vi "MORSE CODE PROJECT COMPLETE.vi"() -> ()   [LabVIEW 2012]
uses:
  <vilib>/Utility/file.llb/Read From Spreadsheet File (string).vi
panel:
  in  "Device Name":tag="Dev1"
  in  "Morse Code Lookup Table File Path":path
  in  "STOP PROGRAM":bool
  in  "Lookup Table":T1
  in  "?":T2(tab)
  out "Telegraph Mode":bool
  out "Light Output":bool
  out "Morse Code Translation":string
  in  "Text Input":string
  in  "Transmit Button":bool
  in  "Dot Speed":dbl(slide) step=5.0 scale=100.0..300.0 scale format="%#_5g"
  in  "RESET TEXT":bool
  out "Translated":string
  out "Waveform Chart":dbl(graph)
  in  "Rate":dbl=1000.0
  in  "Samples":i32=1000
  out "LIVE Decoded Morse Code":string
  in  "Array 2":string[](array[string])
  in  "Array":string[](array[string])
  out "[DEBUG]\nText Indicator":string[](array[string])
  out "[DEBUG]\nIndex of Last Element":i32
  out "[DEBUG] \nMorse Code":string[](array[string])
  out "[DEBUG]\nString":string
  out "Sample Number":dbl
  out "[DEBUG]\nMorse Code Words":string[](array[string])
  in  "Array 3":string[](array[string])
  out "[DEBUG]\nMorse Code Letters":string[](array[string])
  # "Recommended\nSetting:\n\n1. Rate (10000) \n2. Samples (10)"
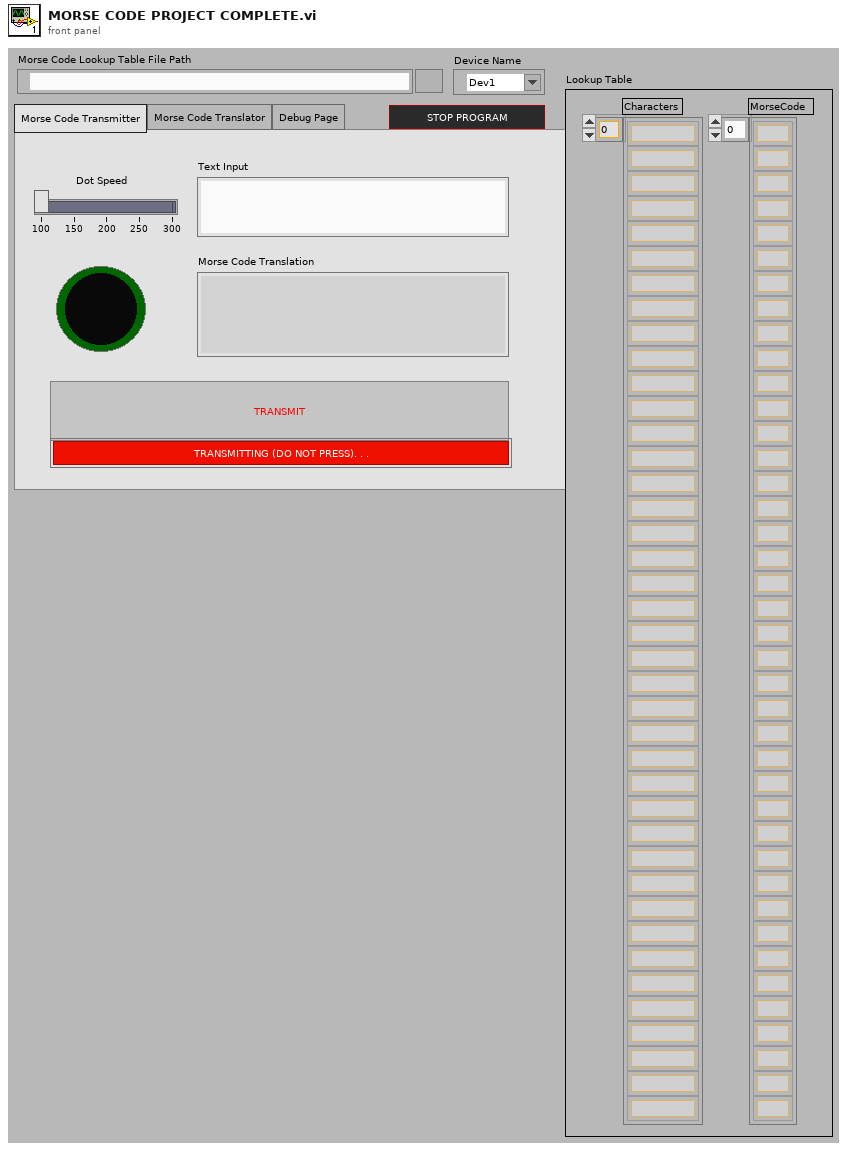
[diagram p1: front panel]
types:
  T1 = cluster{"Characters":string[], "MorseCode":string[]}
  T2 = enum32{"Morse Code Transmitter", "Morse Code Translator", "Debug Page"}
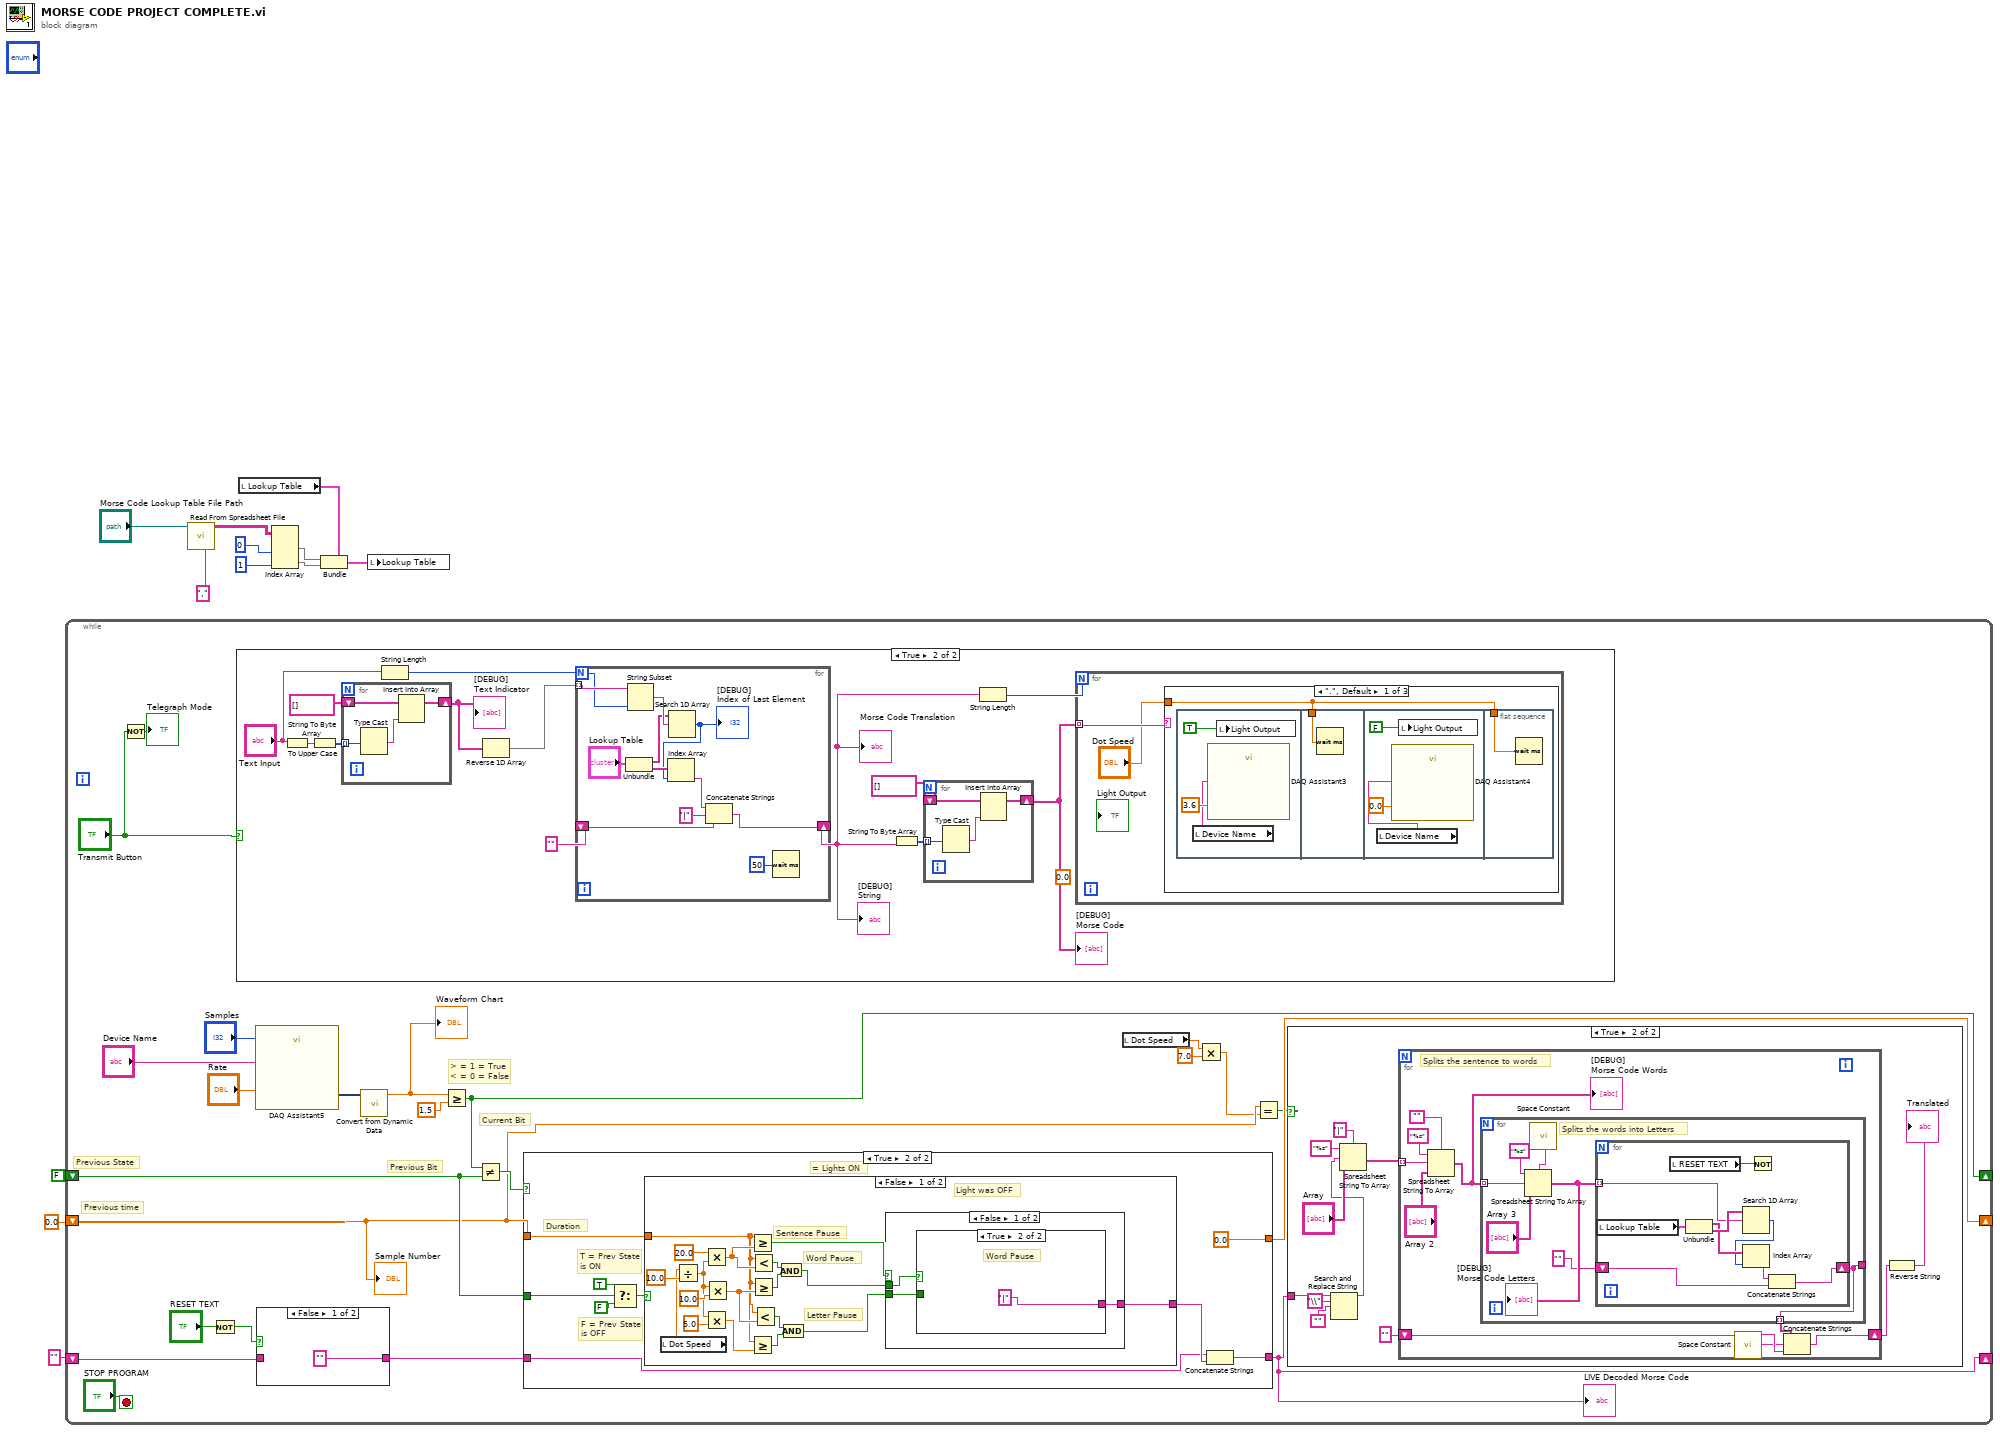
[diagram p0: block diagram]
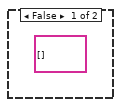
[diagram p2: hidden frame]
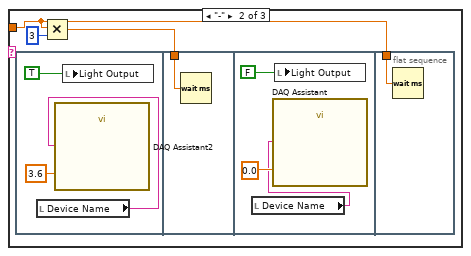
[diagram p5: hidden frame]
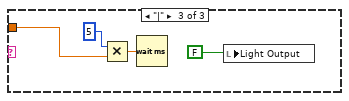
[diagram p6: hidden frame]
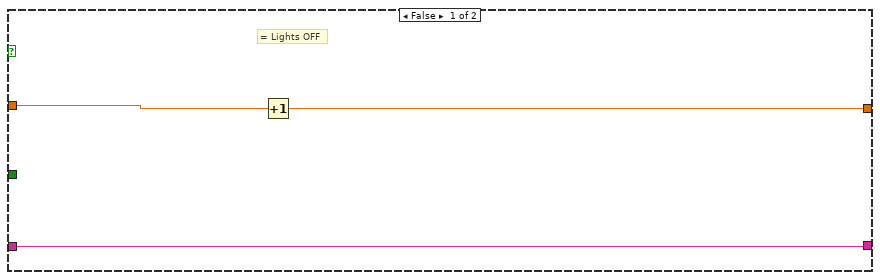
[diagram p7: hidden frame]
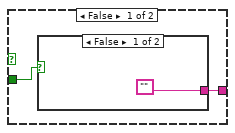
[diagram p8: hidden frame]
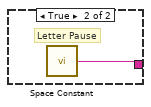
[diagram p9: hidden frame]
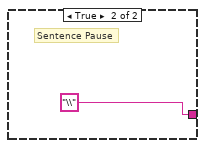
[diagram p10: hidden frame]
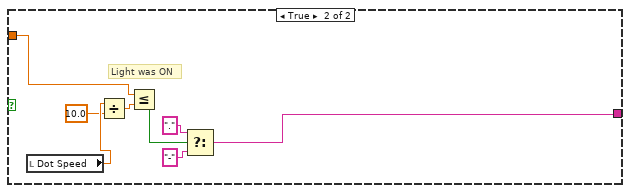
[diagram p11: hidden frame]
diagram:
  n1 = while {
    shift-right: [w29] -> _
    shift-left: FALSE -> [w27]
    shift-right: [w28] -> _
    shift-left: 0.0 -> [w14]
    shift-right: [w18] -> _
    shift-left: "" -> [w21]
    stop <- "STOP PROGRAM" stop-if-true
    # "Previous Bit"
    # "Current Bit"
    # "> = 1 = True\n< = 0 = False"
    # "Previous time"
    # "Previous State"
    n2 = Not(x="Transmit Button") -> (.not. x?=→"Telegraph Mode":bool)
    n3 = Not(x="RESET TEXT") -> (.not. x?=w19:bool)
    n4 = case shown="True" "Transmit Button" {
      frame False {
      }
      frame True {
        (unwired) 0.0
        n5 = To Upper Case(1:"Text Input") -> (0:w84:string)
        n6 = String To Byte Array(string=w84) -> (unsigned byte array=w83:u8[])
        n7 = for {
          tunnel: w83 -> [w120] mode=indexing
          shift-right: [w118] -> w80
          shift-left: string[] [] -> [w119]
          n8 = Type Cast(x=w120) -> (*(type *) &x=w117:string)  [unwired: 1 in]
          n9 = Insert Into Array(array=w119, new element=w117) -> (w118:string[])  [unwired: 1 in]
        }
        "[DEBUG]\nText Indicator" <- w80
        n10 = String Length(string="Text Input") -> (length=w86:i32)
        n11 = Reverse 1D Array(array=w80) -> (reversed array=w81:string[])
        n12 = for {
          N: w86 -> [w125]
          tunnel: w81 -> [w132] mode=indexing
          shift-right: [w122] -> w76
          shift-left: "" -> [w130]
          n13 = Unbundle("Lookup Table") -> ("Characters"=w129:string[], "MorseCode"=w128:string[])
          n14 = String Subset(string=w132, length (rest)=w125) -> (substring=w131:string)  [unwired: 1 in]
          n15 = Search 1D Array(1D array=w129, element=w131) -> (index of element=w124:i32)  [unwired: 1 in]
          "[DEBUG]\nIndex of Last Element" <- w124
          n16 = Index Array(array=w128, index=w124) -> (element=w126:string)
          n17 = Concatenate Strings(w126, "|", w130) -> (w122:string)
          n18 = Wait (ms)(milliseconds to wait=u32 50) -> ()  [unwired: 1 out]
        }
        "Morse Code Translation" <- w76
        "[DEBUG]\nString" <- w76
        n19 = String To Byte Array(string=w76) -> (unsigned byte array=w78:u8[])
        n20 = for {
          tunnel: w78 -> [w116] mode=indexing
          shift-right: [w114] -> w77
          shift-left: string[] [] -> [w115]
          n21 = Type Cast(x=w116) -> (*(type *) &x=w113:string)  [unwired: 1 in]
          n22 = Insert Into Array(array=w115, new element=w113) -> (w114:string[])  [unwired: 1 in]
        }
        "[DEBUG] \nMorse Code" <- w77
        n23 = String Length(string=w76) -> (length=w75:i32)
        n24 = for {
          N: w75 -> [_]
          tunnel: w77 -> [w88] mode=indexing
          n25 = case shown="\".\", Default" w88 {
            tunnel: "Dot Speed" -> [w89 w98 w110]
            frame ".", Default {
              n26 = flat-sequence {
                tunnel: w89 -> [w93]
                tunnel: w89 -> [w97]
                frame #0 {
                  n27 = local read "Device Name"() -> (w90:tag)
                  n28 = call "DAQ Assistant3"("data"=3.6, "device name"=w90) -> ()  [unwired: 16 in, 2 out]
                  n29 = local write "Light Output"(TRUE) -> ()
                }
                frame #1 {
                  n30 = Wait (ms)(milliseconds to wait=w93) -> ()  [unwired: 1 out]
                }
                frame #2 {
                  n31 = local read "Device Name"() -> (w94:tag)
                  n32 = call "DAQ Assistant4"("data"=0.0, "device name"=w94) -> ()  [unwired: 16 in, 2 out]
                  n33 = local write "Light Output"(FALSE) -> ()
                }
                frame #3 {
                  n34 = Wait (ms)(milliseconds to wait=w97) -> ()  [unwired: 1 out]
                }
              }
            }
            frame "-" {
              n35 = flat-sequence {
                tunnel: w99 -> [w104]
                tunnel: w98 -> [w108]
                frame #0 {
                  n36 = local read "Device Name"() -> (w101:tag)
                  n37 = call "DAQ Assistant2"("data"=3.6 ("t"), "device name"=w101) -> ()  [unwired: 16 in, 2 out]
                  n38 = local write "Light Output"(TRUE) -> ()
                }
                frame #1 {
                  n39 = Wait (ms)(milliseconds to wait=w104) -> ()  [unwired: 1 out]
                }
                frame #2 {
                  n40 = local read "Device Name"() -> (w105:tag)
                  n41 = call "DAQ Assistant"("data"=0.0 ("f"), "device name"=w105) -> ()  [unwired: 16 in, 2 out]
                  n42 = local write "Light Output"(FALSE) -> ()
                }
                frame #3 {
                  n43 = Wait (ms)(milliseconds to wait=w108) -> ()  [unwired: 1 out]
                }
              }
              n44 = Multiply(x=w98, y=3) -> (x*y=w99:dbl)
            }
            frame "|" {
              n45 = Multiply(x=5, y=w110) -> (x*y=w112:dbl)
              n46 = Wait (ms)(milliseconds to wait=w112) -> ()  [unwired: 1 out]
              n47 = local write "Light Output"(FALSE ("Time has Elapsed")) -> ()
            }
          }
        }
      }
    }
    n48 = call "DAQ Assistant5"("rate"="Rate", "number of samples"="Samples", "device name"="Device Name") -> ("data"=w31:dynamicdata)  [unwired: 14 in, 2 out]
    n49 = case shown="False" w19 {
      tunnel: w21 -> [_ w73]
      tunnel: ["" w73] -> w22
      frame False {
      }
      frame True {
      }
    }
    n50 = call "Convert from Dynamic Data"("Dynamic Data Type"=w31) -> ("Scalar"=w32:dbl)  [unwired: 3 in]
    "Waveform Chart" <- w32
    n51 = Greater Or Equal?(x=w32, y=1.5) -> (x >= y?=w29:bool)
    n52 = Not Equal?(x=w29, y=w27) -> (x != y?=w30:bool)
    n53 = case shown="True" w30 {
      tunnel: w14 -> [w135 w139]
      tunnel: [w133 0.0] -> w28
      tunnel: w27 -> [_ w144]
      tunnel: [w134 w140] -> w18
      tunnel: w22 -> [w134 w136]
      frame False {
        # "= Lights OFF"
        n54 = Increment(x=w135) -> (x+1=w133:dbl)
      }
      frame True {
        # "F = Prev State\nis OFF"
        # "T = Prev State\nis ON"
        # "Duration"
        # "= Lights ON"
        n55 = Select(t=TRUE, s=w144, f=FALSE) -> (s? t:f=w141:bool)
        n56 = case shown="False" w141 {
          tunnel: [w148 w176] -> w137
          tunnel: w139 -> [w145 w175]
          frame False {
            # "Letter Pause"
            # "Word Pause"
            # "Sentence Pause"
            # "Light was OFF"
            n57 = local read "Dot Speed"() -> (w159:dbl)
            n58 = Divide(x=w159, y=10.0) -> (x/y=w146:dbl)
            n59 = Multiply(x=20.0, y=w146) -> (x*y=w155:dbl)
            n60 = Multiply(x=w146, y=5.0 ("x")) -> (x*y=w153:dbl)
            n61 = Multiply(x=w146, y=10.0 ("x")) -> (x*y=w154:dbl)
            n62 = Greater Or Equal?(x=w145, y=w155) -> (x >= y?=w150:bool)
            n63 = Greater Or Equal?(x=w145, y=w153) -> (x >= y?=w151:bool)
            n64 = Less?(x=w145, y=w155) -> (x < y?=w162:bool)
            n65 = Greater Or Equal?(x=w145, y=w154) -> (x >= y?=w161:bool)
            n66 = Less?(x=w145, y=w154) -> (x < y?=w152:bool)
            n67 = And(x=w162, y=w161) -> (x .and. y?=w149:bool)
            n68 = And(x=w152, y=w151) -> (x .and. y?=w147:bool)
            n69 = case shown="False" w150 {
              tunnel: w149 -> [w165 _]
              tunnel: [w164 "\\"] -> w148
              tunnel: w147 -> [w163 _]
              frame False {
                n70 = case shown="True" w165 {
                  tunnel: [w167 "|"] -> w164
                  tunnel: w163 -> [w166 _]
                  frame False {
                    n71 = case shown="False" w166 {
                      tunnel: ["" w169] -> w167
                      frame False {
                      }
                      frame True {
                        # "Letter Pause"
                        n72 = call <vilib>:"Space Constant.vi"() -> ("String"=w169:string)
                      }
                    }
                  }
                  frame True {
                    # "Word Pause"
                  }
                }
              }
              frame True {
                # "Sentence Pause"
              }
            }
          }
          frame True {
            # "Light was ON"
            n73 = local read "Dot Speed"() -> (w173:dbl)
            n74 = Divide(x=w173, y=10.0) -> (x/y=w174:dbl)
            n75 = Less Or Equal?(x=w175, y=w174) -> (x <= y?=w179:bool)
            n76 = Select(t=".", s=w179, f="-") -> (s? t:f=w176:string)
          }
        }
        n77 = Concatenate Strings(w136, w137) -> (w140:string)
      }
    }
    "LIVE Decoded Morse Code" <- w18
    n78 = local read "Dot Speed"() -> (w16:dbl)
    n79 = Multiply(x=w16, y=7.0 ("x")) -> (x*y=w13:dbl)
    n80 = Equal?(x=w14, y=w13) -> (x = y?=w17:bool)
    n81 = case shown="True" w17 {
      tunnel: w18 -> [_ w42]
      frame False {
        (unwired) string[][] [] ("Array 2")
      }
      frame True {
        n82 = Search and Replace String(input string=w42, search string="\\", replace string="") -> (result string=w39:string)  [unwired: 5 in, 3 out]
        n83 = Spreadsheet String To Array(delimiter (Tab)="|" ("regular expression"), format string="%s", spreadsheet string=w39, array type (2D Dbl)="Array") -> (array=w45:string[])
        n84 = for {
          tunnel: w45 -> [w53] mode=indexing
          shift-right: [w50] -> w38
          shift-left: "" -> [w48]
          # "Splits the sentence to words"
          n85 = Spreadsheet String To Array(delimiter (Tab)="", format string="%s", spreadsheet string=w53, array type (2D Dbl)="Array 2") -> (array=w51:string[])
          "[DEBUG]\nMorse Code Words" <- w51
          n86 = for {
            tunnel: w51 -> [w59] mode=indexing
            tunnel: [w57] -> _
            tunnel: [w57] -> w49 mode=indexing
            # "Splits the words into Letters"
            n87 = call <vilib>:"Space Constant.vi"() -> ("String"=w62:string)
            n88 = Spreadsheet String To Array(delimiter (Tab)=w62, format string="%s", spreadsheet string=w59, array type (2D Dbl)="Array 3") -> (array=w58:string[])
            "[DEBUG]\nMorse Code Letters" <- w58
            n89 = for {
              tunnel: w58 -> [w69] mode=indexing
              shift-right: [w64] -> w57
              shift-left: "" -> [w65]
              n90 = local read "Lookup Table"() -> (w71:T1)
              n91 = local read "RESET TEXT"() -> (w63:bool)
              n92 = Unbundle(w71) -> ("Characters"=w68:string[], "MorseCode"=w70:string[])
              n93 = Search 1D Array(1D array=w70, element=w69) -> (index of element=w67:i32)  [unwired: 1 in]
              n94 = Index Array(array=w68, index=w67) -> (element=w66:string)
              n95 = Not(x=w63) -> ()  [unwired: 1 out]
              n96 = Concatenate Strings(w66, w65) -> (w64:string)
            }
          }
          n97 = call <vilib>:"Space Constant.vi"() -> ("String"=w47:string)
          n98 = Concatenate Strings(w49, w47, w48) -> (w50:string)
        }
        n99 = Reverse String(1:w38) -> (0:→"Translated":string)
      }
    }
    "Sample Number" <- w14
  }
  n100 = call-poly <vilib>:"Read From Spreadsheet File.vi"("delimiter (\\t)"="," ("delimiter (\\t)"), "file path (dialog if empty)"="Morse Code Lookup Table File Path") -> ("all rows"=w9:string[][])  [unwired: 5 in, 4 out]
  n101 = local read "Lookup Table"() -> (w2:T1)
  n102 = Index Array(array=w9, index (col) #1=0 ("index"), index (col) #2=1 ("index")) -> (element #1=w7:string[], element #2=w4:string[])  [unwired: 2 in]
  n103 = Bundle(cluster=w2, "Characters"=w7, "MorseCode"=w4) -> (w3:T1)
  n104 = local write "Lookup Table"(w3) -> ()
